vi "LCDBegin.vi"(8 "error in (no error)":errorcluster, 11 "Baud Rate":u32=9600) -> (0 "error out":errorcluster, 3 "LCDRef":T1)   [LabVIEW 2013]
uses:
  LCDRef.ctl
  <vilib>/Rock Robotics/WPI/SerialPort/WPI_SerialPortRef.ctl
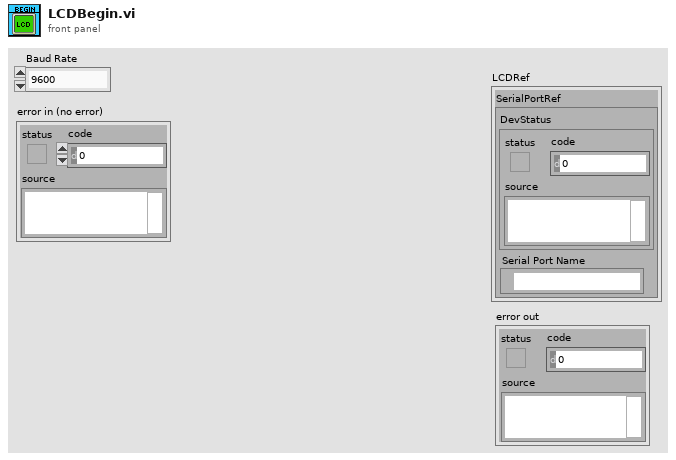
[diagram p1: front panel]
types:
  T1 = typedef "LCDRef.ctl" = cluster{"SerialPortRef":T2}
  T2 = typedef "WPI_SerialPortRef.ctl" = cluster{"DevStatus":errorcluster, "Serial Port Name":refnum<visa-resource-name>}
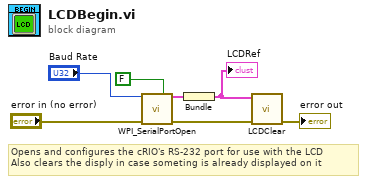
[diagram p0: block diagram]
diagram:
  # "Opens and configures the cRIO's RS-232 port for use with the LCD\nAlso clears the disply in case someting is already displayed on it"
  n1 = call <vilib>:"WPI_SerialPortOpen.vi"("Baud Rate"="Baud Rate", "Enable Termination Char? (T)"=FALSE, "error in (no error)"="error in (no error)") -> ("SerialPortRef"=w4:T2, "error out"=w2:errorcluster)  [unwired: 11 in]
  n2 = Bundle("SerialPortRef"=w4) -> (w3:cluster{"SerialPortRef":T2})  [unwired: 1 in]
  "LCDRef" <- w3
  n3 = call "LCDClear.vi"("error in (no error)"=w2, "LCDRef"=w3) -> ("error out"=→"error out":errorcluster)  [unwired: 9 in]
